vi "auto.vi"() -> ()   [LabVIEW 2010, in "LASA Beta.lvrbt"]
uses:
  LASA Beta.lvrbt
  <vilib>/NXT/Block Support/NXT_ButtonSelector.ctl
  <vilib>/NXT/Dual Mode Library/Display/clearDisplay.vi
  <vilib>/NXT/Dual Mode Library/Display/drawText.vi
  <vilib>/NXT/Dual Mode Library/Sensors/readNXTButton.vi
  <vilib>/NXT/Dual Mode Library/Waits/Wait_Num(msec).vi
  <vilib>/NXT/Dual Mode Library/Display/drawNumber.vi
  op_init.vi
  op_run.vi
  op_read.vi
  <vilib>/NXT/Dual Mode Library/Display/drawNumber_float.vi
panel:
  in  "Speed":dbl=25.0
  in  "Debug Mode":enum16{"DM Off", "DM On"}(ring)
  out "Enabled":bool
  in  "Team Number":string="4290"
  in  "Direction":dbl
  in  "Time Delay":dbl
  in  "Cursor":dbl
  # "INITIALIZATION"
  # "Set this number to display team information"
  # "AUTONOMOUS"
  # "If enabled, use robot is on as read by comm. loop"
  # "Set this to ON to allow the robot to run without communication to the field"
  # "Robot movement speed; slower = more accurate"
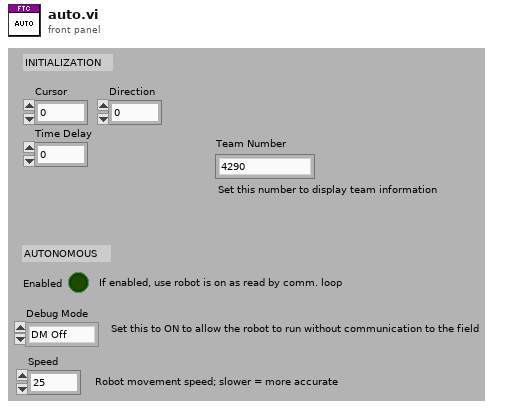
[diagram p1: front panel]
types:
  T1 = typedef "NXT_ButtonSelector.ctl" = u16
  T2 = enum16{"Raise Arm", "Move to Place", "Place Block", "Move Backward", "Lower Arm", "Rotate Left", "Forward to Ramp", "Rotate to Ramp", "Climb Ramp", "Exit"}
  T3 = typedef "LVHSConnector.ctl" = cluster{"Hardware":string, "Flattened String":string}
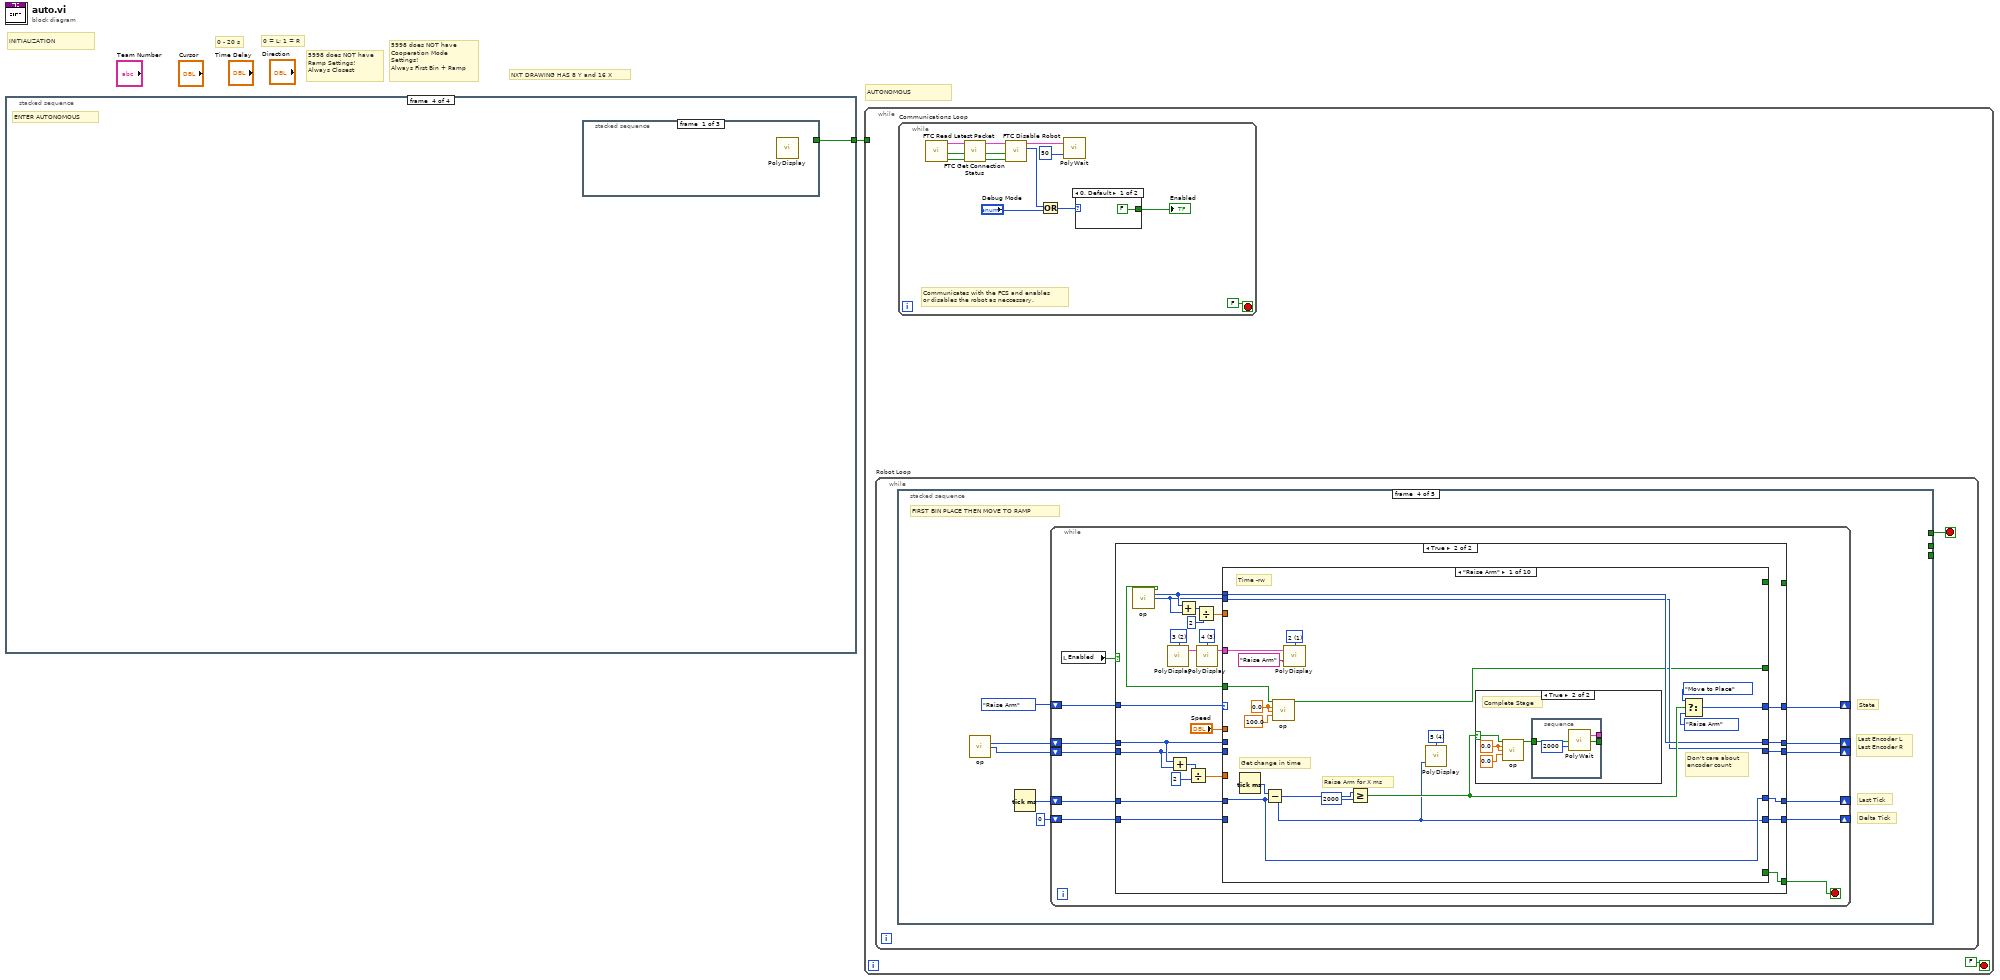
[diagram p0: block diagram]
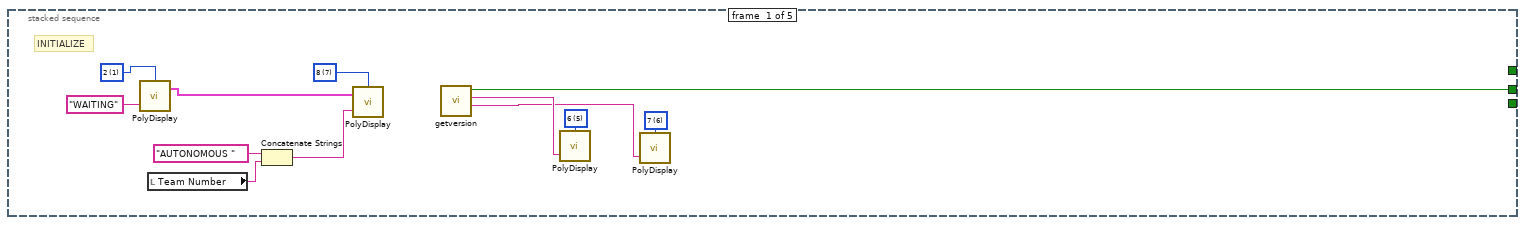
[diagram p2: hidden frame]
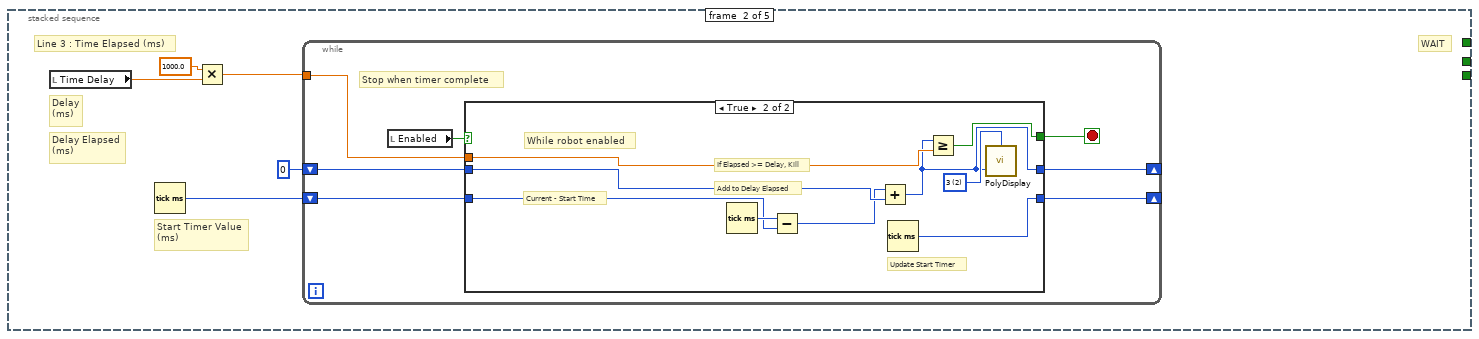
[diagram p3: hidden frame]
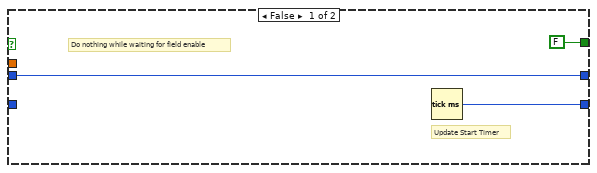
[diagram p4: hidden frame]
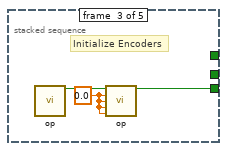
[diagram p5: hidden frame]
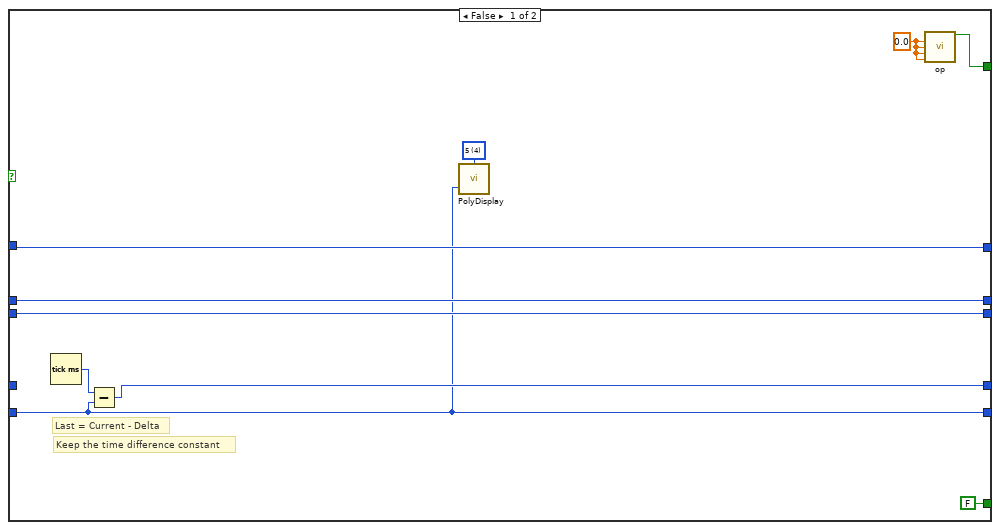
[diagram p6: hidden frame]
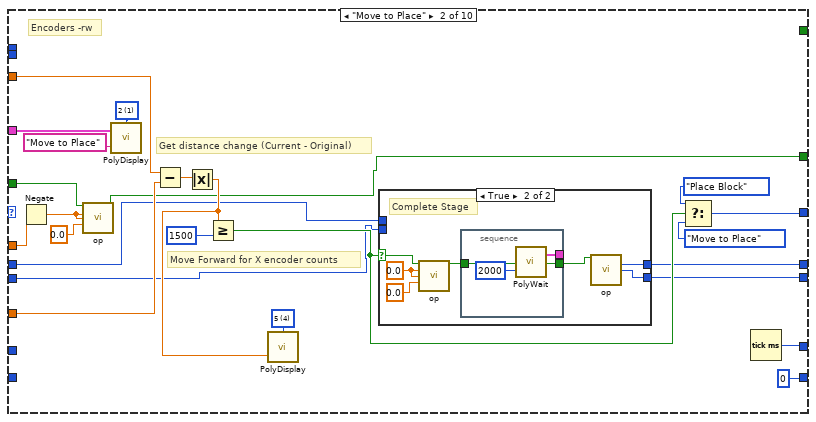
[diagram p8: hidden frame]
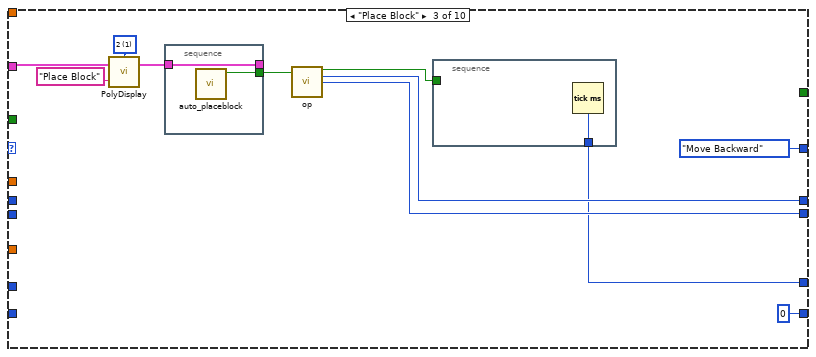
[diagram p10: hidden frame]
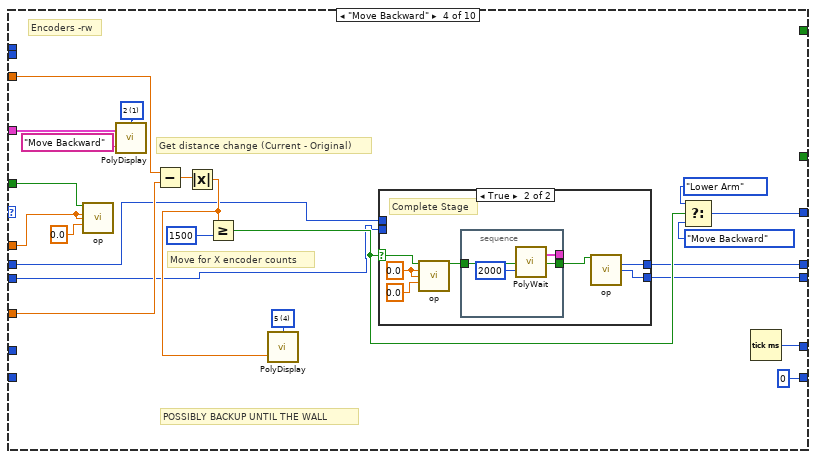
[diagram p11: hidden frame]
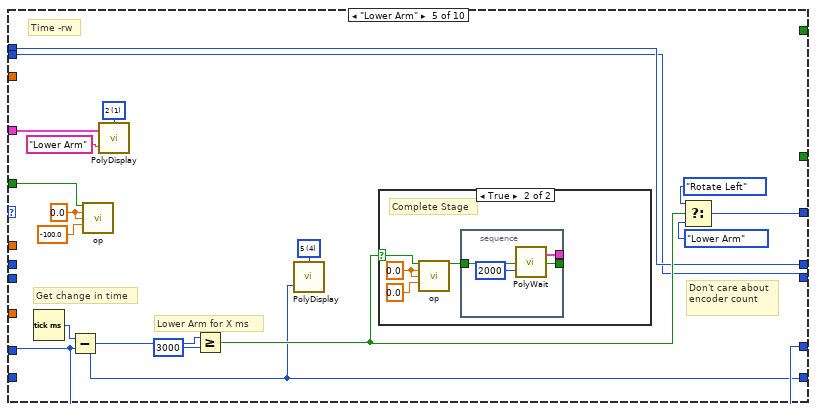
[diagram p13: hidden frame]
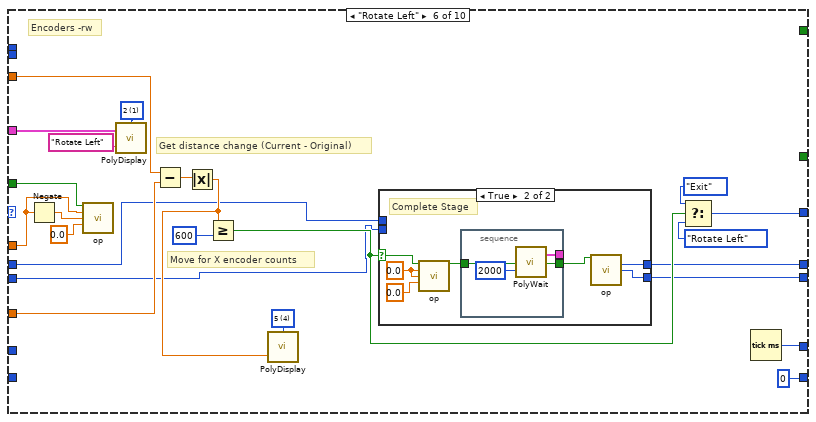
[diagram p15: hidden frame]
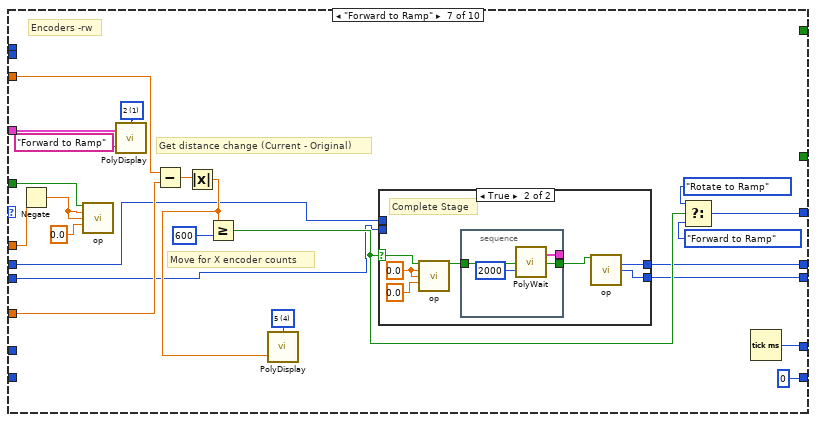
[diagram p17: hidden frame]
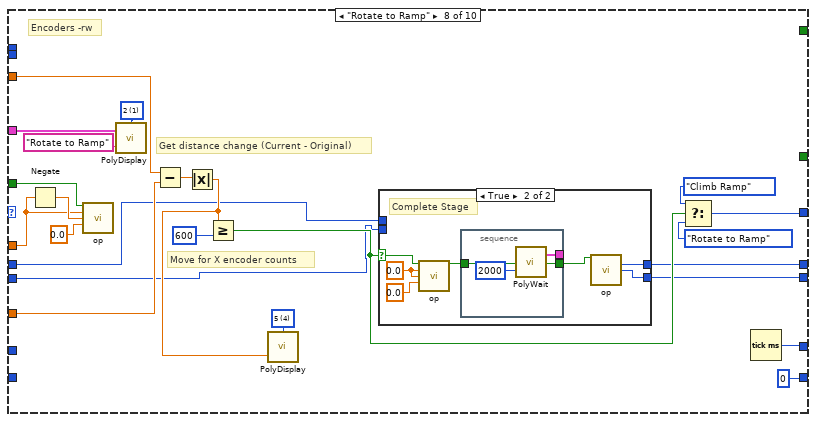
[diagram p19: hidden frame]
diagram:
  # "5998 does NOT have\nCooperation Mode\nSettings!\nAlways First Bin + Ramp"
  # "AUTONOMOUS"
  # "INITIALIZATION"
  # "NXT DRAWING HAS 8 Y and 16 X"
  # "0 = L; 1 = R"
  # "0 - 20 s"
  # "5998 does NOT have\nRamp Settings!\nAlways Closest"
  n1 = stacked-sequence {
    tunnel: [_ _ _ w78] -> w1
    frame #0 {
      # "PREPARE FOR INITIALIZATION"
      n2 = call-poly <vilib>:"PolyDisplay.vi"() -> ()  [unwired: 4 in, 1 out]
    }
    frame #1 {
      n3 = stacked-sequence {
        frame #0 {
          w2 = i16 7 items=["1", "2", "3", "4", "5", "6", "7", "8"] ("Line")
          w10 = i16 2 items=["1", "2", "3", "4", "5", "6", "7", "8"] ("Line")
          w8 = i16 0 items=["1", "2", "3", "4", "5", "6", "7", "8"] ("Line")
          # "-_0 sec_+"
          n4 = local write "Cursor"(0.0 ("Cursor")) -> ()
          n5 = call-poly <vilib>:"PolyDisplay.vi"("Text"="- 0 sec +", "Line"=w10) -> ()  [unwired: 2 in, 1 out]
          n6 = local read "Team Number"() -> (w4:string)
          n7 = call-poly <vilib>:"PolyDisplay.vi"("Text"="TIME DELAY", "Line"=w8) -> ()  [unwired: 2 in, 1 out]
          n8 = Concatenate Strings("AUTONOMOUS " ("string"), w4) -> (w5:string)
          n9 = call-poly <vilib>:"PolyDisplay.vi"("Text"=w5, "Line"=w2) -> ()  [unwired: 2 in, 1 out]
        }
        frame #1 {
          n10 = while {
            stop <- w15 stop-if-true
            w12 = T1 1 items=["Enter button"=3, "Left button"=2, "Right button"=1] ("Button (Enter button)")
            w14 = T1 2 items=["Enter button"=3, "Left button"=2, "Right button"=1] ("Button (Enter button)")
            w17 = T1 3 items=["Enter button"=3, "Left button"=2, "Right button"=1] ("Button (Enter button)")
            n11 = call-poly <vilib>:"PolySensor.vi"("Button (Enter button)"=w14) -> ("Yes/No"=w13:bool)  [unwired: 2 in, 1 out]
            n12 = call-poly <vilib>:"PolySensor.vi"("Button (Enter button)"=w12) -> ("Yes/No"=w11:bool)  [unwired: 2 in, 1 out]
            n13 = call-poly <vilib>:"PolySensor.vi"("Button (Enter button)"=w17) -> ("Yes/No"=w16:bool)  [unwired: 2 in, 1 out]
            n14 = case shown="True" w13 {
              frame False {
              }
              frame True {
                n15 = local read "Cursor"() -> (w40:dbl)
                n16 = Greater?(x=w40, y=0.0) -> (0:w39:bool)
                n17 = case shown="True" w39 {
                  frame False {
                  }
                  frame True {
                    w44 = i16 2 items=["1", "2", "3", "4", "5", "6", "7", "8"] ("Line")
                    n18 = local read "Cursor"() -> (w49:dbl)
                    n19 = Wait (ms)(milliseconds to wait=u32 300) -> ()  [unwired: 1 out]
                    n20 = Subtract(x=w49, y=5.0) -> (x-y=w48:dbl)
                    n21 = local write "Cursor"(w48) -> ()
                    n22 = call <vilib>:"NXT_floatToString.vi"("number"=w48) -> ("string"=w45:string)
                    n23 = Concatenate Strings("- " ("string"), w45, " sec +" ("string")) -> (w43:string)
                    n24 = call-poly <vilib>:"PolyDisplay.vi"("Text"=w43, "Line"=w44) -> ()  [unwired: 2 in, 1 out]
                  }
                }
              }
            }
            n25 = case shown="True" w11 {
              frame False {
              }
              frame True {
                n26 = local read "Cursor"() -> (w20:dbl)
                n27 = Less?(x=w20, y=20.0) -> (x < y?=w18:bool)
                n28 = case shown="True" w18 {
                  frame False {
                  }
                  frame True {
                    w24 = i16 2 items=["1", "2", "3", "4", "5", "6", "7", "8"] ("Line")
                    n29 = local read "Cursor"() -> (w28:dbl)
                    n30 = Wait (ms)(milliseconds to wait=u32 300) -> ()  [unwired: 1 out]
                    n31 = Add(x=w28, y=5.0) -> (x+y=w22:dbl)
                    n32 = local write "Cursor"(w22) -> ()
                    n33 = call <vilib>:"NXT_floatToString.vi"("number"=w22) -> ("string"=w26:string)
                    n34 = Concatenate Strings("- " ("string"), w26, " sec +" ("string")) -> (w25:string)
                    n35 = call-poly <vilib>:"PolyDisplay.vi"("Text"=w25, "Line"=w24) -> ()  [unwired: 2 in, 1 out]
                  }
                }
              }
            }
            n36 = case shown="True" w16 {
              tunnel: [FALSE w31] -> w15
              frame False {
              }
              frame True {
                n37 = stacked-sequence {
                  tunnel: [_ _ TRUE] -> w31
                  frame #0 {
                    n38 = local read "Cursor"() -> (w33:dbl)
                    n39 = local write "Direction"(0.0 ("Direction")) -> ()
                    n40 = local write "Time Delay"(w33) -> ()
                    n41 = call-poly <vilib>:"PolyDisplay.vi"() -> ()  [unwired: 4 in, 1 out]
                  }
                  frame #1 {
                    w36 = i16 0 items=["1", "2", "3", "4", "5", "6", "7", "8"] ("Line")
                    n42 = local write "Cursor"(0.0 ("Cursor")) -> ()
                    n43 = call-poly <vilib>:"PolyDisplay.vi"("Text"="Working...", "Line"=w36) -> ()  [unwired: 2 in, 1 out]
                  }
                  frame #2 {
                    n44 = Wait (ms)(milliseconds to wait=u32 500) -> ()  [unwired: 1 out]
                  }
                }
              }
            }
          }
        }
      }
    }
    frame #2 {
      # "2 = L/R"
      n45 = stacked-sequence {
        frame #0 {
          w51 = i16 3 items=["1", "2", "3", "4", "5", "6", "7", "8"] ("Line")
          w56 = i16 7 items=["1", "2", "3", "4", "5", "6", "7", "8"] ("Line")
          w60 = i16 2 items=["1", "2", "3", "4", "5", "6", "7", "8"] ("Line")
          w58 = i16 0 items=["1", "2", "3", "4", "5", "6", "7", "8"] ("Line")
          n46 = local read "Team Number"() -> (w53:string)
          n47 = call-poly <vilib>:"PolyDisplay.vi"("Text"="[LEFT] = L", "Line"=w60) -> ()  [unwired: 2 in, 1 out]
          n48 = call-poly <vilib>:"PolyDisplay.vi"("Text"="[RIGHT] = R", "Line"=w51) -> ()  [unwired: 2 in, 1 out]
          n49 = Concatenate Strings("AUTONOMOUS " ("string"), w53) -> (w52:string)
          n50 = call-poly <vilib>:"PolyDisplay.vi"("Text"="START LOCATION", "Line"=w58) -> ()  [unwired: 2 in, 1 out]
          n51 = call-poly <vilib>:"PolyDisplay.vi"("Text"=w52, "Line"=w56) -> ()  [unwired: 2 in, 1 out]
        }
        frame #1 {
          n52 = while {
            stop <- w61 stop-if-true
            w66 = T1 1 items=["Enter button"=3, "Left button"=2, "Right button"=1] ("Button (Enter button)")
            w67 = T1 2 items=["Enter button"=3, "Left button"=2, "Right button"=1] ("Button (Enter button)")
            n53 = call-poly <vilib>:"PolySensor.vi"("Button (Enter button)"=w67) -> ("Yes/No"=w64:bool)  [unwired: 2 in, 1 out]
            n54 = call-poly <vilib>:"PolySensor.vi"("Button (Enter button)"=w66) -> ("Yes/No"=w65:bool)  [unwired: 2 in, 1 out]
            n55 = case shown="True" w64 {
              tunnel: [FALSE TRUE] -> w63
              frame False {
              }
              frame True {
                n56 = local write "Direction"(0.0 ("Direction")) -> ()
              }
            }
            n57 = case shown="True" w65 {
              tunnel: [FALSE TRUE] -> w62
              frame False {
              }
              frame True {
                n58 = local write "Direction"(1.0 ("Direction")) -> ()
              }
            }
            n59 = Or(x=w63, y=w62) -> (x .or. y?=w61:bool)
          }
        }
        frame #2 {
          n60 = local write "Cursor"(0.0 ("Cursor")) -> ()
          n61 = call-poly <vilib>:"PolyDisplay.vi"() -> ()  [unwired: 4 in, 1 out]
        }
        frame #3 {
          w76 = i16 0 items=["1", "2", "3", "4", "5", "6", "7", "8"] ("Line")
          n62 = call-poly <vilib>:"PolyDisplay.vi"("Text"="Working...", "Line"=w76) -> ()  [unwired: 2 in, 1 out]
        }
        frame #4 {
          n63 = Wait (ms)(milliseconds to wait=u32 500) -> ()  [unwired: 1 out]
        }
      }
    }
    frame #3 {
      # "ENTER AUTONOMOUS"
      n64 = stacked-sequence {
        tunnel: [_ _ FALSE] -> w78
        frame #0 {
          n65 = call-poly <vilib>:"PolyDisplay.vi"() -> ()  [unwired: 4 in, 1 out]
        }
        frame #1 {
          w82 = i16 7 items=["1", "2", "3", "4", "5", "6", "7", "8"] ("Line")
          n66 = local read "Team Number"() -> (w79:string)
          n67 = Concatenate Strings("AUTONOMOUS " ("string"), w79) -> (w80:string)
          n68 = call-poly <vilib>:"PolyDisplay.vi"("Text"=w80, "Line"=w82) -> ()  [unwired: 2 in, 1 out]
        }
        frame #2 {
        }
      }
    }
  }
  n69 = while {
    tunnel: w1 -> [_]
    stop <- FALSE stop-if-true
    n70 = while "Robot Loop" {
      stop <- w85 stop-if-true
      n71 = stacked-sequence {
        tunnel: [_ _ _ _ TRUE] -> w85
        tunnel: [_ _ w122 _ _] -> _
        tunnel: [w90 _ _ _ _] -> _
        frame #0 {
          w87 = i16 6 items=["1", "2", "3", "4", "5", "6", "7", "8"] ("Line")
          w89 = i16 5 items=["1", "2", "3", "4", "5", "6", "7", "8"] ("Line")
          w95 = i16 7 items=["1", "2", "3", "4", "5", "6", "7", "8"] ("Line")
          w97 = i16 1 items=["1", "2", "3", "4", "5", "6", "7", "8"] ("Line")
          # "INITIALIZE"
          n72 = call-poly <vilib>:"PolyDisplay.vi"("Text"="WAITING", "Line"=w97) -> ("NXT"=w91:T3)  [unwired: 2 in]
          n73 = local read "Team Number"() -> (w93:string)
          n74 = Concatenate Strings("AUTONOMOUS " ("string"), w93) -> (w92:string)
          n75 = call-poly <vilib>:"PolyDisplay.vi"("Text"=w92, "NXT"=w91, "Line"=w95) -> ()  [unwired: 1 in, 1 out]
          n76 = call "getversion.vi"() -> ("Revision"=w86:string, "Version"=w88:string, "Chain OUT"=w90:bool)  [unwired: 9 in]
          n77 = call-poly <vilib>:"PolyDisplay.vi"("Text"=w88, "Line"=w89) -> ()  [unwired: 2 in, 1 out]
          n78 = call-poly <vilib>:"PolyDisplay.vi"("Text"=w86, "Line"=w87) -> ()  [unwired: 2 in, 1 out]
        }
        frame #1 {
          # "Line 3 : Time Elapsed (ms)"
          # "Delay\n(ms)"
          # "Start Timer Value\n(ms)"
          # "Delay Elapsed\n(ms)"
          # "WAIT"
          n79 = local read "Time Delay"() -> (w101:dbl)
          n80 = Tick Count (ms)() -> (millisecond timer value=w98:u32)
          n81 = Multiply(x=1000.0, y=w101) -> (x*y=w99:dbl)
          n82 = while {
            shift-right: [w103] -> _
            shift-left: 0 -> [w106]
            tunnel: w99 -> [w108]
            shift-right: [w105] -> _
            shift-left: w98 -> [w107]
            stop <- w104 stop-if-true
            # "Stop when timer complete"
            n83 = local read "Enabled"() -> (w109:bool)
            n84 = case shown="True" w109 {
              tunnel: w108 -> [_ w117]
              tunnel: w107 -> [_ w118]
              tunnel: w106 -> [w111 w120]
              tunnel: [w112 w115] -> w105
              tunnel: [FALSE w116] -> w104
              tunnel: [w111 w113] -> w103
              frame False {
                # "Do nothing while waiting for field enable"
                # "Update Start Timer"
                n85 = Tick Count (ms)() -> (millisecond timer value=w112:u32)
              }
              frame True {
                w114 = i16 2 items=["1", "2", "3", "4", "5", "6", "7", "8"] ("Line")
                # "Update Start Timer"
                # "If Elapsed >= Delay, Kill"
                # "Add to Delay Elapsed"
                # "Current - Start Time"
                # "While robot enabled"
                n86 = Tick Count (ms)() -> (millisecond timer value=w121:u32)
                n87 = Subtract(x=w121, y=w118) -> (x-y=w119:u32)
                n88 = Add(x=w119, y=w120) -> (x+y=w113:u32)
                n89 = Tick Count (ms)() -> (millisecond timer value=w115:u32)
                n90 = Greater Or Equal?(x=w113, y=w117) -> (x >= y?=w116:bool)
                n91 = call-poly <vilib>:"PolyDisplay.vi"("number"=w113, "Line"=w114) -> ()  [unwired: 2 in, 1 out]
              }
            }
          }
        }
        frame #2 {
          w123 = 0.0 ("Left Drive")
          # "Initialize Encoders"
          n92 = call-poly "op.vi"() -> ("Chain OUT"=w124:bool)  [unwired: 15 in]
          n93 = call-poly "op.vi"("Chain IN"=w124, "Left Drive"=w123, "Right Drive"=w123, "Arm Control"=w123, "Lift String Control"=w123) -> ("Chain OUT"=w122:bool)  [unwired: 10 in]
        }
        frame #3 {
          # "Delta Tick"
          # "Last Tick"
          # "Last Encoder L Last Encoder R"
          # "State"
          # "FIRST BIN PLACE THEN MOVE TO RAMP"
          n94 = call-poly "op.vi"() -> ("Encoder Left Drive"=w126:i32, "Encoder Right Drive"=w125:i32)  [unwired: 11 in, 3 out]
          n95 = Tick Count (ms)() -> (millisecond timer value=w128:u32)
          n96 = while {
            shift-right: [w137] -> _
            shift-left: T2."Raise Arm" -> [w139]
            shift-right: [w135] -> _
            shift-left: w128 -> [w138]
            shift-right: [w130] -> _
            shift-left: u32 0 -> [w136]
            shift-right: [w134] -> _
            shift-left: w126 -> [w133]
            shift-right: [w132] -> _
            shift-left: w125 -> [w131]
            stop <- w140 stop-if-true
            n97 = local read "Enabled"() -> (w141:bool)
            n98 = case shown="True" w141 {
              tunnel: [FALSE w173] -> w140
              tunnel: w139 -> [w149 w176]
              tunnel: w138 -> [_ w172]
              tunnel: [w149 w170] -> w137
              tunnel: [w148 _] -> _
              tunnel: [w142 w169] -> w130
              tunnel: w136 -> [w142 w158]
              tunnel: [w144 w168] -> w135
              tunnel: [w147 w160] -> w134
              tunnel: w133 -> [w147 w156]
              tunnel: w131 -> [w146 w155]
              tunnel: [w146 w159] -> w132
              frame False {
                w143 = i16 4 items=["1", "2", "3", "4", "5", "6", "7", "8"] ("Line")
                w151 = 0.0 ("Left Drive")
                # "Last = Current - Delta"
                # "Keep the time difference constant"
                n99 = Tick Count (ms)() -> (millisecond timer value=w145:u32)
                n100 = Subtract(x=w145, y=w142) -> (x-y=w144:u32)
                n101 = call-poly <vilib>:"PolyDisplay.vi"("number"=w142, "Line"=w143) -> ()  [unwired: 2 in, 1 out]
                n102 = call-poly "op.vi"("Left Drive"=w151, "Right Drive"=w151, "Arm Control"=w151, "Lift String Control"=w151) -> ("Chain OUT"=w148:bool)  [unwired: 11 in]
              }
              frame True {
                w174 = i16 3 items=["1", "2", "3", "4", "5", "6", "7", "8"] ("Line")
                w175 = i16 2 items=["1", "2", "3", "4", "5", "6", "7", "8"] ("Line")
                n103 = call-poly "op.vi"() -> ("Chain OUT"=w166:bool, "Encoder Left Drive"=w165:i32, "Encoder Right Drive"=w164:i32)  [unwired: 11 in, 2 out]
                n104 = call-poly <vilib>:"PolyDisplay.vi"("Line"=w175) -> ("NXT"=w167:T3)  [unwired: 3 in]
                n105 = Add(x=w156, y=w155) -> (x+y=w154:i32)
                n106 = Add(x=w165, y=w164) -> (x+y=w163:i32)
                n107 = Divide(x=w154, y=2) -> (x/y=w152:dbl)
                n108 = Divide(x=w163, y=2) -> (x/y=w161:dbl)
                n109 = call-poly <vilib>:"PolyDisplay.vi"("NXT"=w167, "Line"=w174) -> ("NXT"=w171:T3)  [unwired: 2 in]
                n110 = case shown="\"Raise Arm\"" w176 {
                  tunnel: [_ _ _ _ _ _ _ _ _ TRUE] -> w173
                  tunnel: w172 -> [w184 _ _ _ w292 _ _ _ _ _]
                  tunnel: w171 -> [w192 w224 w246 w272 w300 w331 w366 w401 w436 w450]
                  tunnel: [w187 w219 T2."Move Backward" w267 w295 w326 w361 w396 w431 _] -> w170
                  tunnel: [w177 u32 0 u32 0 u32 0 w286 u32 0 u32 0 u32 0 u32 0 _] -> w169
                  tunnel: [w184 w214 w239 w262 w292 w321 w356 w391 w426 _] -> w168
                  tunnel: w166 -> [w182 w216 _ w264 w290 w323 w358 w393 w428 _]
                  tunnel: w165 -> [w181 _ _ _ w289 _ _ _ _ _]
                  tunnel: w164 -> [w180 _ _ _ w288 _ _ _ _ _]
                  tunnel: w161 -> [_ w212 _ w260 _ w319 w354 w389 w424 _]
                  tunnel: [w181 w206 w243 w254 w289 w313 w348 w383 w418 _] -> w160
                  tunnel: [w180 w205 w242 w253 w288 w312 w347 w382 w417 _] -> w159
                  tunnel: w156 -> [_ w208 _ w256 _ w315 w350 w385 w420 _]
                  tunnel: [_ _ _ _ _ _ _ _ _ w454] -> _
                  tunnel: w158 -> [_ _ _ _ _ _ _ _ _ _]
                  tunnel: w155 -> [_ w207 _ w255 _ w314 w349 w384 w419 _]
                  tunnel: "Speed" -> [_ w204 _ w252 _ w311 w346 w380 w416 _]
                  tunnel: w152 -> [_ w211 _ w259 _ w318 w353 w388 w423 _]
                  tunnel: [w179 w203 _ _ _ _ _ _ _ _] -> _
                  frame "Raise Arm" {
                    w178 = i16 4 items=["1", "2", "3", "4", "5", "6", "7", "8"] ("Line")
                    w191 = i16 1 items=["1", "2", "3", "4", "5", "6", "7", "8"] ("Line")
                    w194 = 0.0 ("Left Drive")
                    # "Don't care about\nencoder count"
                    # "Get change in time"
                    # "Time -rw"
                    # "Raise Arm for X ms"
                    n111 = Tick Count (ms)() -> (millisecond timer value=w186:u32)
                    n112 = Subtract(x=w186, y=w184) -> (x-y=w177:u32)
                    n113 = call-poly "op.vi"("Chain IN"=w182, "Left Drive"=w194, "Right Drive"=w194, "Arm Control"=100.0) -> ("Chain OUT"=w179:bool)  [unwired: 11 in]
                    n114 = call-poly <vilib>:"PolyDisplay.vi"("Text"="Raise Arm", "NXT"=w192, "Line"=w191) -> ()  [unwired: 1 in, 1 out]
                    n115 = Greater Or Equal?(x=w177, y=u32 2000) -> (x >= y?=w183:bool)
                    n116 = call-poly <vilib>:"PolyDisplay.vi"("number"=w177, "Line"=w178) -> ()  [unwired: 2 in, 1 out]
                    n117 = case shown="True" w183 {
                      selector: w183 -> [_ w195]
                      frame False {
                      }
                      frame True {
                        w198 = 0.0 ("Left Drive")
                        # "Complete Stage"
                        n118 = call-poly "op.vi"("Chain IN"=w195, "Left Drive"=w198, "Right Drive"=w198, "Arm Control"=0.0) -> ("Chain OUT"=w196:bool)  [unwired: 11 in]
                        n119 = stacked-sequence {
                          tunnel: w196 -> [w199]
                          tunnel: [w200] -> _
                          tunnel: [w199] -> _
                          frame #0 {
                            n120 = call-poly <vilib>:"PolyWait.vi"("Time (100 msec)"=u32 2000) -> ("NXT"=w200:T3)  [unwired: 3 in]
                          }
                        }
                      }
                    }
                    n121 = Select(t=T2."Move to Place", s=w183, f=T2."Raise Arm") -> (s? t:f=w187:T2)
                  }
                  frame "Move to Place" {
                    w210 = i16 4 items=["1", "2", "3", "4", "5", "6", "7", "8"] ("Line")
                    w223 = i16 1 items=["1", "2", "3", "4", "5", "6", "7", "8"] ("Line")
                    # "Get distance change (Current - Original)"
                    # "Encoders -rw"
                    # "Move Forward for X encoder counts"
                    n122 = Negate(x=w204) -> (-x=w202:dbl)
                    n123 = call-poly "op.vi"("Chain IN"=w216, "Left Drive"=w202, "Right Drive"=w202, "Arm Control"=0.0) -> ("Chain OUT"=w203:bool)  [unwired: 11 in]
                    n124 = call-poly <vilib>:"PolyDisplay.vi"("Text"="Move to Place", "NXT"=w224, "Line"=w223) -> ()  [unwired: 1 in, 1 out]
                    n125 = Subtract(x=w212, y=w211) -> (x-y=w213:dbl)
                    n126 = Absolute Value(x=w213) -> (abs(x)=w209:dbl)
                    n127 = Greater Or Equal?(x=w209, y=u32 1500) -> (x >= y?=w217:bool)
                    n128 = call-poly <vilib>:"PolyDisplay.vi"("number"=w209, "Line"=w210) -> ()  [unwired: 2 in, 1 out]
                    n129 = case shown="True" w217 {
                      selector: w217 -> [_ w231]
                      tunnel: w208 -> [w227 _]
                      tunnel: w207 -> [w226 _]
                      tunnel: [w227 w229] -> w206
                      tunnel: [w226 w228] -> w205
                      frame False {
                      }
                      frame True {
                        w234 = 0.0 ("Left Drive")
                        # "Complete Stage"
                        n130 = call-poly "op.vi"("Chain IN"=w231, "Left Drive"=w234, "Right Drive"=w234, "Arm Control"=0.0) -> ("Chain OUT"=w232:bool)  [unwired: 11 in]
                        n131 = stacked-sequence {
                          tunnel: w232 -> [w235]
                          tunnel: [w236] -> _
                          tunnel: [w235] -> w230
                          frame #0 {
                            n132 = call-poly <vilib>:"PolyWait.vi"("Time (100 msec)"=u32 2000) -> ("NXT"=w236:T3)  [unwired: 3 in]
                          }
                        }
                        n133 = call-poly "op.vi"("Chain IN"=w230) -> ("Encoder Left Drive"=w229:i32, "Encoder Right Drive"=w228:i32)  [unwired: 10 in, 3 out]
                      }
                    }
                    n134 = Select(t=T2."Place Block", s=w217, f=T2."Move to Place") -> (s? t:f=w219:T2)
                    n135 = Tick Count (ms)() -> (millisecond timer value=w214:u32)
                  }
                  frame "Place Block" {
                    w248 = i16 1 items=["1", "2", "3", "4", "5", "6", "7", "8"] ("Line")
                    n136 = call-poly <vilib>:"PolyDisplay.vi"("Text"="Place Block", "NXT"=w246, "Line"=w248) -> ("NXT"=w245:T3)  [unwired: 1 in]
                    n137 = stacked-sequence {
                      tunnel: w245 -> [w250]
                      tunnel: [w251] -> w244
                      tunnel: [w250] -> _
                      frame #0 {
                        n138 = call "auto_placeblock.vi"() -> ("Chain OUT"=w251:bool)  [unwired: 11 in]
                      }
                    }
                    n139 = call-poly "op.vi"("Chain IN"=w244) -> ("Chain OUT"=w241:bool, "Encoder Left Drive"=w243:i32, "Encoder Right Drive"=w242:i32)  [unwired: 10 in, 2 out]
                    n140 = stacked-sequence {
                      tunnel: w241 -> [_]
                      tunnel: [w249] -> w239
                      frame #0 {
                        n141 = Tick Count (ms)() -> (millisecond timer value=w249:u32)
                      }
                    }
                  }
                  frame "Move Backward" {
                    w258 = i16 4 items=["1", "2", "3", "4", "5", "6", "7", "8"] ("Line")
                    w271 = i16 1 items=["1", "2", "3", "4", "5", "6", "7", "8"] ("Line")
                    # "POSSIBLY BACKUP UNTIL THE WALL"
                    # "Get distance change (Current - Original)"
                    # "Encoders -rw"
                    # "Move for X encoder counts"
                    n142 = call-poly "op.vi"("Chain IN"=w264, "Left Drive"=w252, "Right Drive"=w252, "Arm Control"=0.0) -> ()  [unwired: 11 in, 1 out]
                    n143 = call-poly <vilib>:"PolyDisplay.vi"("Text"="Move Backward", "NXT"=w272, "Line"=w271) -> ()  [unwired: 1 in, 1 out]
                    n144 = Subtract(x=w260, y=w259) -> (x-y=w261:dbl)
                    n145 = Absolute Value(x=w261) -> (abs(x)=w257:dbl)
                    n146 = Greater Or Equal?(x=w257, y=u32 1500) -> (x >= y?=w265:bool)
                    n147 = call-poly <vilib>:"PolyDisplay.vi"("number"=w257, "Line"=w258) -> ()  [unwired: 2 in, 1 out]
                    n148 = case shown="True" w265 {
                      selector: w265 -> [_ w279]
                      tunnel: w256 -> [w275 _]
                      tunnel: w255 -> [w274 _]
                      tunnel: [w275 w277] -> w254
                      tunnel: [w274 w276] -> w253
                      frame False {
                      }
                      frame True {
                        w282 = 0.0 ("Left Drive")
                        # "Complete Stage"
                        n149 = call-poly "op.vi"("Chain IN"=w279, "Left Drive"=w282, "Right Drive"=w282, "Arm Control"=0.0) -> ("Chain OUT"=w280:bool)  [unwired: 11 in]
                        n150 = stacked-sequence {
                          tunnel: w280 -> [w283]
                          tunnel: [w284] -> _
                          tunnel: [w283] -> w278
                          frame #0 {
                            n151 = call-poly <vilib>:"PolyWait.vi"("Time (100 msec)"=u32 2000) -> ("NXT"=w284:T3)  [unwired: 3 in]
                          }
                        }
                        n152 = call-poly "op.vi"("Chain IN"=w278) -> ("Encoder Left Drive"=w277:i32, "Encoder Right Drive"=w276:i32)  [unwired: 10 in, 3 out]
                      }
                    }
                    n153 = Select(t=T2."Lower Arm", s=w265, f=T2."Move Backward") -> (s? t:f=w267:T2)
                    n154 = Tick Count (ms)() -> (millisecond timer value=w262:u32)
                  }
                  frame "Lower Arm" {
                    w287 = i16 4 items=["1", "2", "3", "4", "5", "6", "7", "8"] ("Line")
                    w299 = i16 1 items=["1", "2", "3", "4", "5", "6", "7", "8"] ("Line")
                    w302 = 0.0 ("Left Drive")
                    # "Don't care about\nencoder count"
                    # "Get change in time"
                    # "Time -rw"
                    # "Lower Arm for X ms"
                    n155 = Tick Count (ms)() -> (millisecond timer value=w294:u32)
                    n156 = Subtract(x=w294, y=w292) -> (x-y=w286:u32)
                    n157 = call-poly "op.vi"("Chain IN"=w290, "Left Drive"=w302, "Right Drive"=w302, "Arm Control"=-100.0) -> ()  [unwired: 11 in, 1 out]
                    n158 = call-poly <vilib>:"PolyDisplay.vi"("Text"="Lower Arm", "NXT"=w300, "Line"=w299) -> ()  [unwired: 1 in, 1 out]
                    n159 = Greater Or Equal?(x=w286, y=u32 3000) -> (x >= y?=w291:bool)
                    n160 = call-poly <vilib>:"PolyDisplay.vi"("number"=w286, "Line"=w287) -> ()  [unwired: 2 in, 1 out]
                    n161 = case shown="True" w291 {
                      selector: w291 -> [_ w303]
                      frame False {
                      }
                      frame True {
                        w306 = 0.0 ("Left Drive")
                        # "Complete Stage"
                        n162 = call-poly "op.vi"("Chain IN"=w303, "Left Drive"=w306, "Right Drive"=w306, "Arm Control"=0.0) -> ("Chain OUT"=w304:bool)  [unwired: 11 in]
                        n163 = stacked-sequence {
                          tunnel: w304 -> [w307]
                          tunnel: [w308] -> _
                          tunnel: [w307] -> _
                          frame #0 {
                            n164 = call-poly <vilib>:"PolyWait.vi"("Time (100 msec)"=u32 2000) -> ("NXT"=w308:T3)  [unwired: 3 in]
                          }
                        }
                      }
                    }
                    n165 = Select(t=T2."Rotate Left", s=w291, f=T2."Lower Arm") -> (s? t:f=w295:T2)
                  }
                  frame "Rotate Left" {
                    w317 = i16 4 items=["1", "2", "3", "4", "5", "6", "7", "8"] ("Line")
                    w330 = i16 1 items=["1", "2", "3", "4", "5", "6", "7", "8"] ("Line")
                    # "Get distance change (Current - Original)"
                    # "Encoders -rw"
                    # "Move for X encoder counts"
                    n166 = Negate(x=w311) -> (-x=w310:dbl)
                    n167 = call-poly "op.vi"("Chain IN"=w323, "Left Drive"=w311, "Right Drive"=w310, "Arm Control"=0.0) -> ()  [unwired: 11 in, 1 out]
                    n168 = call-poly <vilib>:"PolyDisplay.vi"("Text"="Rotate Left", "NXT"=w331, "Line"=w330) -> ()  [unwired: 1 in, 1 out]
                    n169 = Subtract(x=w319, y=w318) -> (x-y=w320:dbl)
                    n170 = Absolute Value(x=w320) -> (abs(x)=w316:dbl)
                    n171 = Greater Or Equal?(x=w316, y=u32 600) -> (x >= y?=w324:bool)
                    n172 = call-poly <vilib>:"PolyDisplay.vi"("number"=w316, "Line"=w317) -> ()  [unwired: 2 in, 1 out]
                    n173 = case shown="True" w324 {
                      selector: w324 -> [_ w338]
                      tunnel: w315 -> [w334 _]
                      tunnel: w314 -> [w333 _]
                      tunnel: [w334 w336] -> w313
                      tunnel: [w333 w335] -> w312
                      frame False {
                      }
                      frame True {
                        w341 = 0.0 ("Left Drive")
                        # "Complete Stage"
                        n174 = call-poly "op.vi"("Chain IN"=w338, "Left Drive"=w341, "Right Drive"=w341, "Arm Control"=0.0) -> ("Chain OUT"=w339:bool)  [unwired: 11 in]
                        n175 = stacked-sequence {
                          tunnel: w339 -> [w342]
                          tunnel: [w343] -> _
                          tunnel: [w342] -> w337
                          frame #0 {
                            n176 = call-poly <vilib>:"PolyWait.vi"("Time (100 msec)"=u32 2000) -> ("NXT"=w343:T3)  [unwired: 3 in]
                          }
                        }
                        n177 = call-poly "op.vi"("Chain IN"=w337) -> ("Encoder Left Drive"=w336:i32, "Encoder Right Drive"=w335:i32)  [unwired: 10 in, 3 out]
                      }
                    }
                    n178 = Select(t=T2."Exit", s=w324, f=T2."Rotate Left") -> (s? t:f=w326:T2)
                    n179 = Tick Count (ms)() -> (millisecond timer value=w321:u32)
                  }
                  frame "Forward to Ramp" {
                    w352 = i16 4 items=["1", "2", "3", "4", "5", "6", "7", "8"] ("Line")
                    w365 = i16 1 items=["1", "2", "3", "4", "5", "6", "7", "8"] ("Line")
                    # "Get distance change (Current - Original)"
                    # "Encoders -rw"
                    # "Move for X encoder counts"
                    n180 = Negate(x=w346) -> (-x=w345:dbl)
                    n181 = call-poly "op.vi"("Chain IN"=w358, "Left Drive"=w345, "Right Drive"=w345, "Arm Control"=0.0) -> ()  [unwired: 11 in, 1 out]
                    n182 = call-poly <vilib>:"PolyDisplay.vi"("Text"="Forward to Ramp", "NXT"=w366, "Line"=w365) -> ()  [unwired: 1 in, 1 out]
                    n183 = Subtract(x=w354, y=w353) -> (x-y=w355:dbl)
                    n184 = Absolute Value(x=w355) -> (abs(x)=w351:dbl)
                    n185 = Greater Or Equal?(x=w351, y=u32 600) -> (x >= y?=w359:bool)
                    n186 = call-poly <vilib>:"PolyDisplay.vi"("number"=w351, "Line"=w352) -> ()  [unwired: 2 in, 1 out]
                    n187 = case shown="True" w359 {
                      selector: w359 -> [_ w373]
                      tunnel: w350 -> [w369 _]
                      tunnel: w349 -> [w368 _]
                      tunnel: [w369 w371] -> w348
                      tunnel: [w368 w370] -> w347
                      frame False {
                      }
                      frame True {
                        w376 = 0.0 ("Left Drive")
                        # "Complete Stage"
                        n188 = call-poly "op.vi"("Chain IN"=w373, "Left Drive"=w376, "Right Drive"=w376, "Arm Control"=0.0) -> ("Chain OUT"=w374:bool)  [unwired: 11 in]
                        n189 = stacked-sequence {
                          tunnel: w374 -> [w377]
                          tunnel: [w378] -> _
                          tunnel: [w377] -> w372
                          frame #0 {
                            n190 = call-poly <vilib>:"PolyWait.vi"("Time (100 msec)"=u32 2000) -> ("NXT"=w378:T3)  [unwired: 3 in]
                          }
                        }
                        n191 = call-poly "op.vi"("Chain IN"=w372) -> ("Encoder Left Drive"=w371:i32, "Encoder Right Drive"=w370:i32)  [unwired: 10 in, 3 out]
                      }
                    }
                    n192 = Select(t=T2."Rotate to Ramp", s=w359, f=T2."Forward to Ramp") -> (s? t:f=w361:T2)
                    n193 = Tick Count (ms)() -> (millisecond timer value=w356:u32)
                  }
                  frame "Rotate to Ramp" {
                    w387 = i16 4 items=["1", "2", "3", "4", "5", "6", "7", "8"] ("Line")
                    w400 = i16 1 items=["1", "2", "3", "4", "5", "6", "7", "8"] ("Line")
                    # "Get distance change (Current - Original)"
                    # "Encoders -rw"
                    # "Move for X encoder counts"
                    n194 = Negate(x=w380) -> (-x=w381:dbl)
                    n195 = call-poly "op.vi"("Chain IN"=w393, "Left Drive"=w380, "Right Drive"=w381, "Arm Control"=0.0) -> ()  [unwired: 11 in, 1 out]
                    n196 = call-poly <vilib>:"PolyDisplay.vi"("Text"="Rotate to Ramp", "NXT"=w401, "Line"=w400) -> ()  [unwired: 1 in, 1 out]
                    n197 = Subtract(x=w389, y=w388) -> (x-y=w390:dbl)
                    n198 = Absolute Value(x=w390) -> (abs(x)=w386:dbl)
                    n199 = Greater Or Equal?(x=w386, y=u32 600) -> (x >= y?=w394:bool)
                    n200 = call-poly <vilib>:"PolyDisplay.vi"("number"=w386, "Line"=w387) -> ()  [unwired: 2 in, 1 out]
                    n201 = case shown="True" w394 {
                      selector: w394 -> [_ w408]
                      tunnel: w385 -> [w404 _]
                      tunnel: w384 -> [w403 _]
                      tunnel: [w404 w406] -> w383
                      tunnel: [w403 w405] -> w382
                      frame False {
                      }
                      frame True {
                        w411 = 0.0 ("Left Drive")
                        # "Complete Stage"
                        n202 = call-poly "op.vi"("Chain IN"=w408, "Left Drive"=w411, "Right Drive"=w411, "Arm Control"=0.0) -> ("Chain OUT"=w409:bool)  [unwired: 11 in]
                        n203 = stacked-sequence {
                          tunnel: w409 -> [w412]
                          tunnel: [w413] -> _
                          tunnel: [w412] -> w407
                          frame #0 {
                            n204 = call-poly <vilib>:"PolyWait.vi"("Time (100 msec)"=u32 2000) -> ("NXT"=w413:T3)  [unwired: 3 in]
                          }
                        }
                        n205 = call-poly "op.vi"("Chain IN"=w407) -> ("Encoder Left Drive"=w406:i32, "Encoder Right Drive"=w405:i32)  [unwired: 10 in, 3 out]
                      }
                    }
                    n206 = Select(t=T2."Climb Ramp", s=w394, f=T2."Rotate to Ramp") -> (s? t:f=w396:T2)
                    n207 = Tick Count (ms)() -> (millisecond timer value=w391:u32)
                  }
                  frame "Climb Ramp" {
                    w422 = i16 4 items=["1", "2", "3", "4", "5", "6", "7", "8"] ("Line")
                    w435 = i16 1 items=["1", "2", "3", "4", "5", "6", "7", "8"] ("Line")
                    # "Get distance change (Current - Original)"
                    # "Encoders -rw"
                    # "Move for X encoder counts"
                    n208 = Negate(x=w416) -> (-x=w415:dbl)
                    n209 = call-poly "op.vi"("Chain IN"=w428, "Left Drive"=w415, "Right Drive"=w415, "Arm Control"=0.0) -> ()  [unwired: 11 in, 1 out]
                    n210 = call-poly <vilib>:"PolyDisplay.vi"("Text"="Climb Ramp", "NXT"=w436, "Line"=w435) -> ()  [unwired: 1 in, 1 out]
                    n211 = Subtract(x=w424, y=w423) -> (x-y=w425:dbl)
                    n212 = Absolute Value(x=w425) -> (abs(x)=w421:dbl)
                    n213 = Greater Or Equal?(x=w421, y=u32 600) -> (x >= y?=w429:bool)
                    n214 = call-poly <vilib>:"PolyDisplay.vi"("number"=w421, "Line"=w422) -> ()  [unwired: 2 in, 1 out]
                    n215 = case shown="True" w429 {
                      selector: w429 -> [_ w443]
                      tunnel: w420 -> [w439 _]
                      tunnel: w419 -> [w438 _]
                      tunnel: [w439 w441] -> w418
                      tunnel: [w438 w440] -> w417
                      frame False {
                      }
                      frame True {
                        w446 = 0.0 ("Left Drive")
                        # "Complete Stage"
                        n216 = call-poly "op.vi"("Chain IN"=w443, "Left Drive"=w446, "Right Drive"=w446, "Arm Control"=0.0) -> ("Chain OUT"=w444:bool)  [unwired: 11 in]
                        n217 = stacked-sequence {
                          tunnel: w444 -> [w447]
                          tunnel: [w448] -> _
                          tunnel: [w447] -> w442
                          frame #0 {
                            n218 = call-poly <vilib>:"PolyWait.vi"("Time (100 msec)"=u32 2000) -> ("NXT"=w448:T3)  [unwired: 3 in]
                          }
                        }
                        n219 = call-poly "op.vi"("Chain IN"=w442) -> ("Encoder Left Drive"=w441:i32, "Encoder Right Drive"=w440:i32)  [unwired: 10 in, 3 out]
                      }
                    }
                    n220 = Select(t=T2."Exit", s=w429, f=T2."Climb Ramp") -> (s? t:f=w431:T2)
                    n221 = Tick Count (ms)() -> (millisecond timer value=w426:u32)
                  }
                  frame "Exit", Default {
                    w452 = i16 1 items=["1", "2", "3", "4", "5", "6", "7", "8"] ("Line")
                    w455 = 0.0 ("Left Drive")
                    n222 = call-poly <vilib>:"PolyDisplay.vi"("Text"="Exit", "NXT"=w450, "Line"=w452) -> ()  [unwired: 1 in, 1 out]
                    n223 = call-poly "op.vi"("Left Drive"=w455, "Right Drive"=w455, "Arm Control"=w455, "Lift String Control"=w455) -> ("Chain OUT"=w454:bool)  [unwired: 11 in]
                  }
                }
              }
            }
          }
        }
        frame #4 {
          w457 = 0.0 ("Left Drive")
          w459 = i16 1 items=["1", "2", "3", "4", "5", "6", "7", "8"] ("Line")
          # "KILL LOOP"
          n224 = call-poly <vilib>:"PolyDisplay.vi"("Text"="COMPLETE!", "Line"=w459) -> ()  [unwired: 2 in, 1 out]
          n225 = call-poly "op.vi"("Dump Control"=128.0, "Left Drive"=w457, "Right Drive"=w457, "Arm Control"=w457, "Lift String Control"=w457) -> ()  [unwired: 10 in, 1 out]
        }
      }
    }
    n226 = while "Communications Loop" {
      stop <- FALSE stop-if-true
      # "Communicates with the FCS and enables \nor disables the robot as neccessary."
      n227 = call <vilib>:"FTC Read Latest Packet.vi"() -> ("Packet Received?"=w471:bool, "Stopped?"=w470:bool, "NXT"=w473:T3)  [unwired: 6 in, 3 out]
      n228 = call <vilib>:"FTC Get Connection Status.vi"("Packet Received?"=w471, "Stopped?"=w470, "NXT"=w473) -> ("Online?"=w465:bool, "Stopped?"=w466:bool, "NXT"=w472:T3)  [unwired: 5 in]
      n229 = call <vilib>:"FTC Disable Robot.vi"("Online?"=w465, "Stopped?"=w466, "NXT"=w472) -> ("Enabled?"=w464:enum16{"Disabled", "Enabled"}, "NXT"=w468:T3)  [unwired: 3 in]
      n230 = Or(x=w464, y="Debug Mode") -> (x .or. y?=w463:u16)
      n231 = call-poly <vilib>:"PolyWait.vi"("Time (100 msec)"=u32 50 ("Time (msec)"), "NXT"=w468) -> ()  [unwired: 2 in, 1 out]
      n232 = case shown="0, Default" w463 {
        tunnel: [FALSE TRUE] -> w462
        frame 0, Default {
        }
        frame 1 {
        }
      }
      "Enabled" <- w462
    }
  }
